vi "Load Time and Cycles.vi"(8 "error in (no error)":errorcluster, 11 "Attributes in":refnum<class "Attributes.lvclass">) -> (0 "error out":errorcluster, 2 "Wash Complete":bool, 3 "Attributes out":refnum<class "Attributes.lvclass">)   [LabVIEW 2021, in "Attributes.lvclass"]
uses:
  Attributes.lvclass
  Attributes.lvclass/Attributes.ctl
panel:
  out "Time to Perform":u32
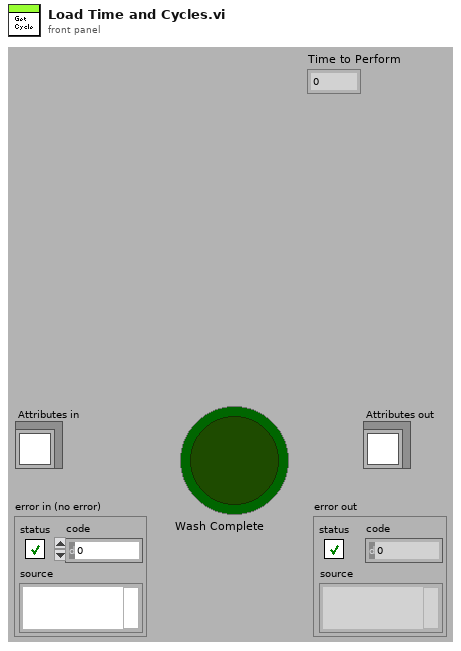
[diagram p1: front panel]
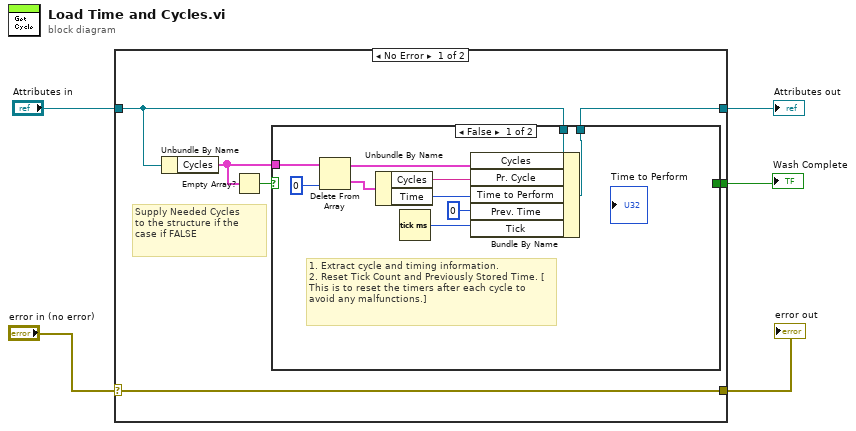
[diagram p0: block diagram]
diagram:
  n1 = case shown="No Error" "error in (no error)" {
    selector: "error in (no error)" -> [w11 w25]
    tunnel: [w11 w25] -> w4
    tunnel: [w9 w24] -> w2
    tunnel: "Attributes in" -> [w10 w24]
    tunnel: [w6 _] -> w1
    frame No Error {
      # "Supply Needed Cycles\nto the structure if the \ncase if FALSE"
      n2 = Unbundle By Name(w10) -> ("Cycles"=w7:cluster{"Cycles":string, "Time":u32}[])
      n3 = Empty Array?(array=w7) -> (empty?=w8:bool)
      n4 = case shown="False" w8 {
        selector: w8 -> [_ w22]
        tunnel: w10 -> [w21 w23]
        tunnel: [w20 w23] -> w9
        tunnel: w7 -> [w19 _]
        tunnel: [_ w22] -> w6
        frame False {
          # "1. Extract cycle and timing information.\n2. Reset Tick Count and Previously Stored Time. [ This is to reset the timers after each cycle to avoid any malfunctions.]"
          n5 = Delete From Array(array=w19, index=0) -> (deleted portion=w17:cluster{"Cycles":string, "Time":u32}, array with subset deleted=w14:cluster{"Cycles":string, "Time":u32}[])  [unwired: 1 in]
          n6 = Unbundle By Name(w17) -> ("Cycles"=w16:string, "Time"=w15:u32)
          n7 = Tick Count (ms)() -> (millisecond timer value=w12:u32)
          n8 = Bundle By Name(cluster=w21, "Cycles"=w14, "Pr. Cycle"=w16, "Time to Perform"=w15, "Prev. Time"=u32 0, "Tick"=w12) -> (w20:refnum<class "Attributes.lvclass">)
        }
        frame True {
          # ">>All Cycles Complete>>"
          # "This section confirms the completion of the  wash sequence and promts the main VI to enable the wash-type selection again."
        }
      }
    }
    frame Error {
    }
  }
  "error out" <- w4
  "Attributes out" <- w2
  "Wash Complete" <- w1
